vi "Update Controller State.vi"(8 "error in (no error)":errorcluster, 11 "Elevator Controller Actor in":refnum<class "Elevator Controller Actor.lvclass">) -> (0 "error out":errorcluster, 3 "Elevator Controller Actor out":refnum<class "Elevator Controller Actor.lvclass">)   [LabVIEW 2019, in "Elevator Controller Actor.lvlib" / "Elevator Controller Actor.lvclass"]
uses:
  Elevator Controller Actor.lvclass
  <vilib>/ActorFramework/Actor/Actor.lvclass
  Sim Display Console Actor/Elevator Controller/Elevator Direction.ctl
  Sim Display Console Actor/Elevator Controller/Sim Display Console Actor.lvclass
  Elevator Controller Actor Messages/Set State Msg/Set State Msg.lvclass
  State -Enum.ctl
  Sim User Console Actor/Elevator Controller/Floor Selection.ctl
  Sim User Console Actor/Elevator Controller/Sim User Console Actor.lvclass
  Sim User Console Actor/Elevator Controller/Elevator Call.ctl
  Sim Display Console Actor/Elevator Controller/Floor -Enum.ctl
  Configuration Database Actor/Configuration Database Actor Messages/Read Record(sec) Msg/Read Record(sec) Msg.lvclass
  Configuration Database Actor/Configuration Database Actor Messages/Write Record(sec) Msg/Write Record(sec) Msg.lvclass
  <vilib>/ActorFramework/Message Enqueuer/Message Enqueuer.lvclass
  Configuration Database Actor/Configuration Database Actor/Record -Cluster.ctl
  Configuration Database Actor/Configuration Database Actor/Configuration Database Actor.lvclass
  Sim Display Console Actor/Sim Display Console Actor Messages/Read value elevator location Msg/Read value elevator location Msg.lvclass
  Sim Display Console Actor/Sim Display Console Actor Messages/Write Timing Msg/Write Timing Msg.lvclass
  Sim User Console Actor/Sim User Console Actor Messages/Disable Doors Msg/Disable Doors Msg.lvclass
  Simulated Sensor Interface Actor/Sim Sensor Interface Messages/Write Elevator Position Msg/Write Elevator Position Msg.lvclass
  Sim Display Console Actor/Sim Display Console Actor Messages/Write Elevator Location Msg/Write Elevator Location Msg.lvclass
  Sim Display Console Actor/Sim Display Console Actor Messages/Write Elevator Direction Msg/Write Elevator Direction Msg.lvclass
  Sim Display Console Actor/Sim Display Console Actor Messages/Write Door Open Msg/Write Door Open Msg.lvclass
  Sim Display Console Actor/Sim Display Console Actor Messages/Write Emergency Ind Msg/Write Emergency Ind Msg.lvclass
  Sim User Console Actor/Sim User Console Actor Messages/Write Elevator Call Msg/Write Elevator Call Msg.lvclass
  Sim User Console Actor/Sim User Console Actor Messages/Write Doors Msg/Write Doors Msg.lvclass
  Sim User Console Actor/Elevator Controller/Door Buttons.ctl
  Sim User Console Actor/Sim User Console Actor Messages/Write Floor Selection Msg/Write Floor Selection Msg.lvclass
  Sim User Console Actor/Sim User Console Actor Messages/Write Emergency Msg/Write Emergency Msg.lvclass
  Sim User Console Actor/Sim User Console Actor Messages/Read all Controls Msg/Read all Controls Msg.lvclass
  Sim Display Console Actor/Sim Display Console Actor Messages/Read Elevator Direction Msg/Read Elevator Direction Msg.lvclass
  Elevator Controller Actor Messages/Set Enable Door Msg/Set Enable Door Msg.lvclass
  Sim User Console Actor/Sim User Console Actor Messages/Disable All components Msg/Disable All components Msg.lvclass
  C:/Program Files (x86)/National Instruments/LabVIEW 2019/vi.lib/ActorFramework/Actor/Actor.lvclass
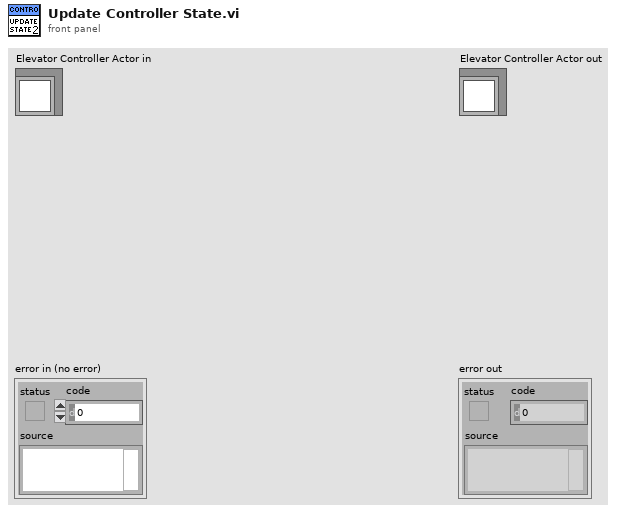
[diagram p1: front panel]
types:
  T1 = typedef "Simulated User Console Actor.lvlib/Sim User Console Actor.lvclass/Floor Selection.ctl" = cluster{"Floor4":bool, "Floor 3":bool, "Floor2":bool, "Floor1":bool}
  T2 = typedef "Simulated User Console Actor.lvlib/Sim User Console Actor.lvclass/Door Buttons.ctl" = cluster{"Open Door":bool, "Close Door":bool}
  T3 = typedef "Simulated User Console Actor.lvlib/Sim User Console Actor.lvclass/Elevator Call.ctl" = cluster{"Up":bool, "Up 2":bool, "Up 3":bool, "Down":bool, "Down 2":bool, "Down 3":bool}
  T4 = typedef "Simulated Display Console Actor.lvlib/Sim Display Console Actor.lvclass/Elevator Direction.ctl" = cluster{"Up":bool, "Down":bool}
  T5 = typedef "Simulated Display Console Actor.lvlib/Sim Display Console Actor.lvclass/Floor -Enum.ctl" = enum16{"First Floor", "Send Floor", "Third Floor", "Fourth Floor"}
  T6 = typedef "Configuration Database Actor.lvlib/Configuration Database Actor.lvclass/Record -Cluster.ctl" = cluster{"Door Open":dbl, "Door close":dbl, "Travel Time":dbl, "Inactive Time":dbl}
  T7 = enum8{"Enabled", "Disabled", "Disabled and Grayed Out"}
  T8 = typedef "Elevator Controller Actor.lvlib/Elevator Controller Actor.lvclass/State -Enum.ctl" = enum16{"Initial", "Wait for First Request", "Start and Move", "Anaysis", "Continue Travel", "Stop at Floor", "Open and Close Door Sequence", "No Request Remaining", "Emergency Call", "Terminate Process"}
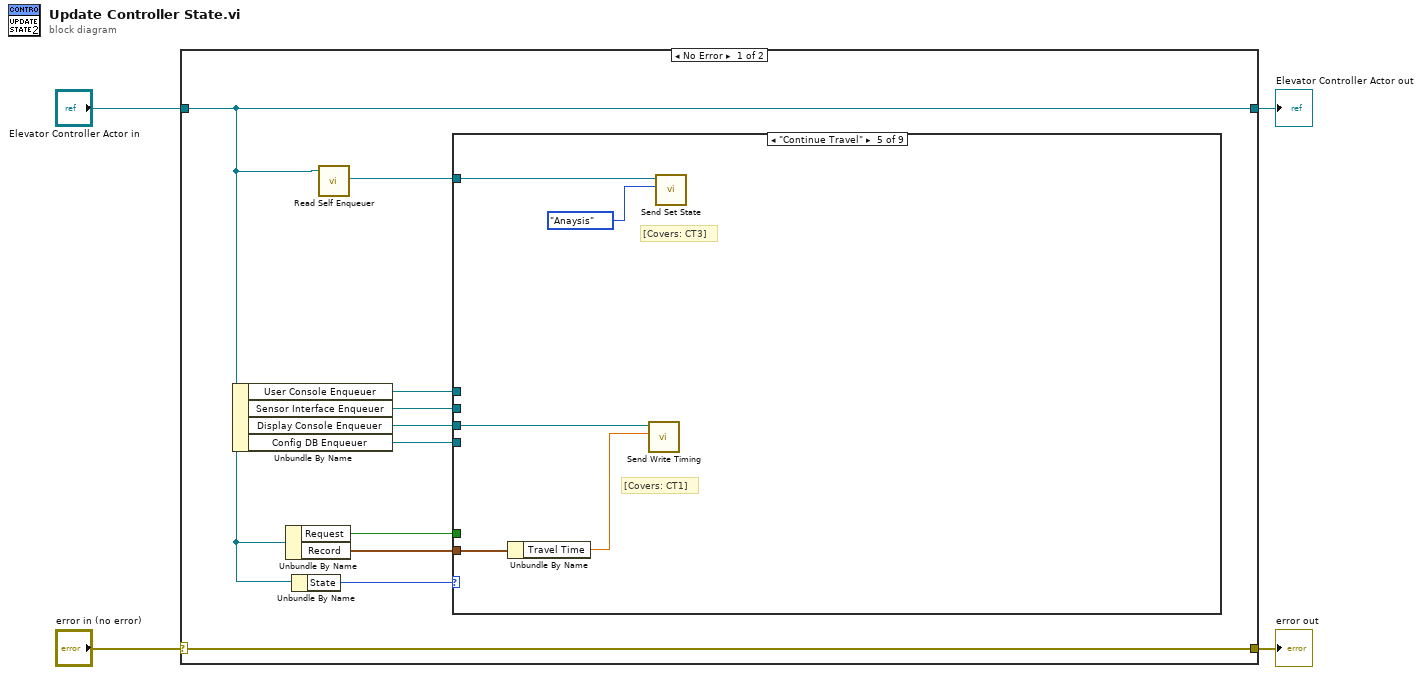
[diagram p0: block diagram]
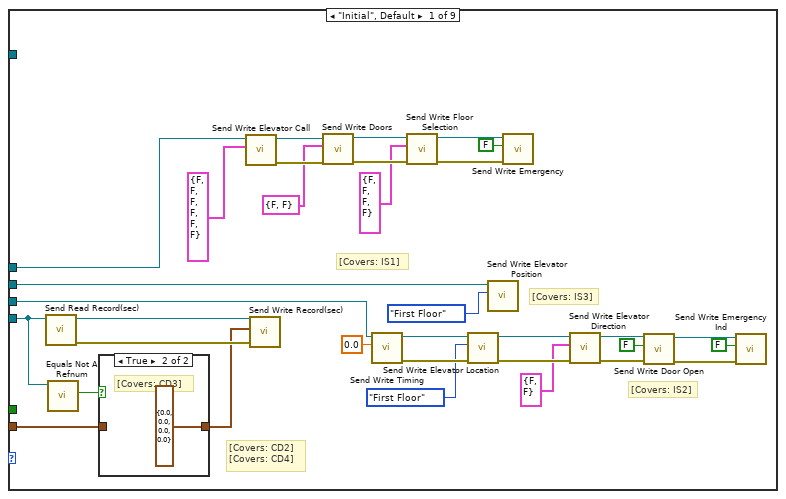
[diagram p2: hidden frame]
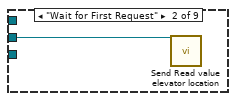
[diagram p4: hidden frame]
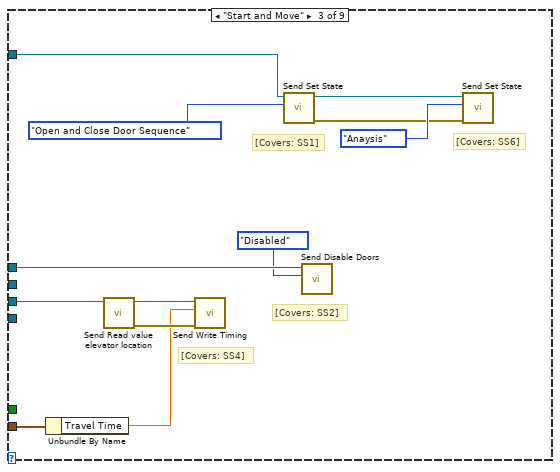
[diagram p5: hidden frame]
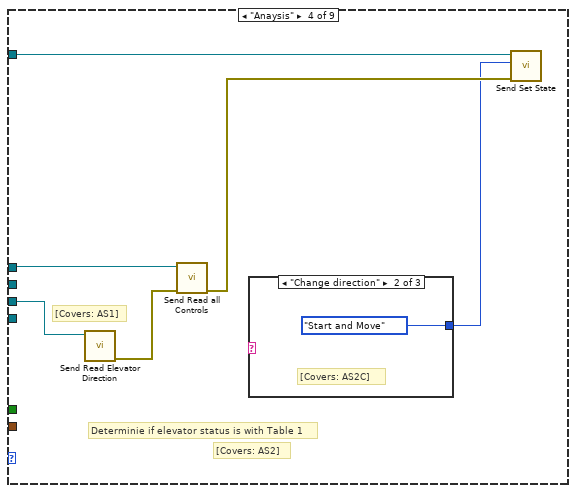
[diagram p6: hidden frame]
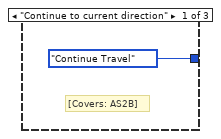
[diagram p7: hidden frame]
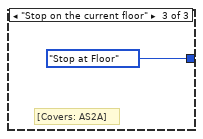
[diagram p8: hidden frame]
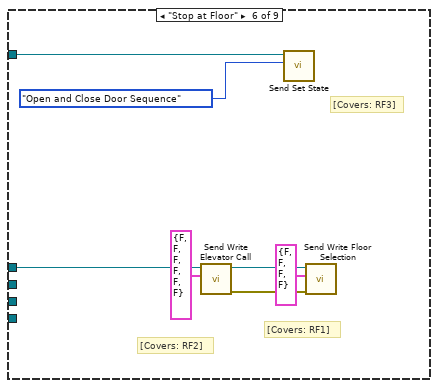
[diagram p9: hidden frame]
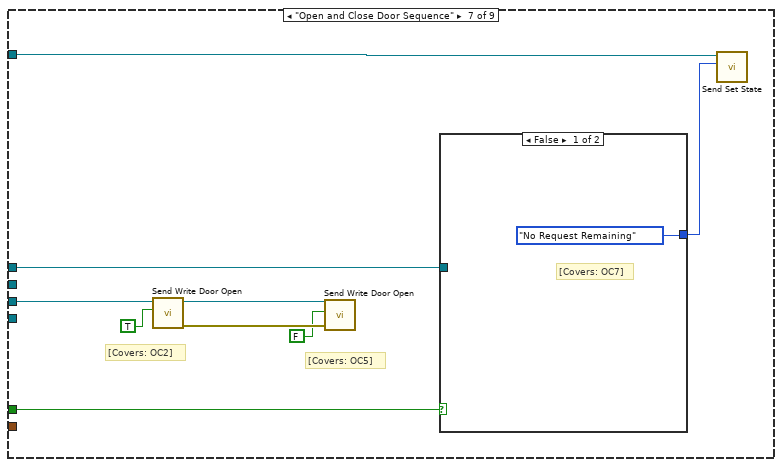
[diagram p10: hidden frame]
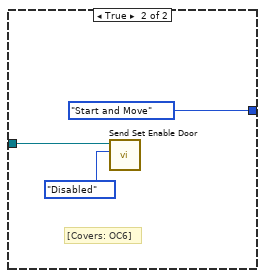
[diagram p11: hidden frame]
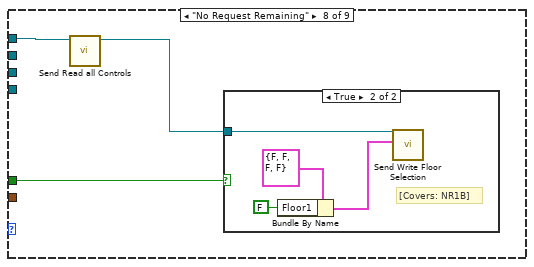
[diagram p12: hidden frame]
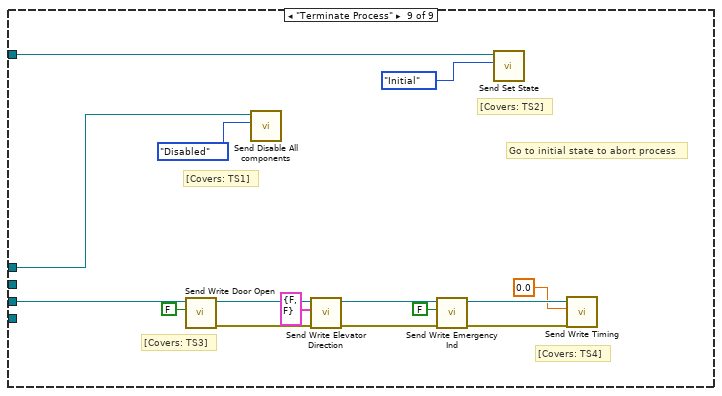
[diagram p14: hidden frame]
diagram:
  n1 = case shown="No Error" "error in (no error)" {
    selector: "error in (no error)" -> [w14 w120]
    tunnel: [w14 w120] -> w3
    tunnel: [w10 w119] -> w1
    tunnel: "Elevator Controller Actor in" -> [w10 w119]
    frame No Error {
      n2 = Unbundle By Name(w10) -> ("User Console Enqueuer"=w6:refnum<class "Message Enqueuer.lvclass">, "Sensor Interface Enqueuer"=w7:refnum<class "Message Enqueuer.lvclass">, "Display Console Enqueuer"=w8:refnum<class "Message Enqueuer.lvclass">, "Config DB Enqueuer"=w11:refnum<class "Message Enqueuer.lvclass">)
      n3 = Unbundle By Name(w10) -> ("Request"=w5:bool, "Record"=w9:T6)
      n4 = Unbundle By Name(w10) -> ("State"=w13:T8)
      n5 = call <vilib>:"Read Self Enqueuer.vi"("Actor"=w10) -> ("Self Enqueuer"=w12:refnum<class "Message Enqueuer.lvclass">)  [unwired: 10 in]
      n6 = case shown="\"Continue Travel\"" w13 {
        tunnel: w12 -> [_ _ w61 w65 w75 w83 w92 _ w105]
        tunnel: w11 -> [w45 _ _ _ _ _ _ _ _]
        tunnel: w9 -> [w43 _ w57 _ w74 _ _ _ _]
        tunnel: w8 -> [w39 w50 w58 w67 w73 _ w91 _ w116]
        tunnel: w7 -> [w40 _ _ _ _ _ _ _ _]
        tunnel: w6 -> [w25 _ w52 w68 _ w79 w85 w98 w118]
        tunnel: w5 -> [_ _ _ _ _ _ w86 w99 _]
        frame "Initial", Default {
          # "[Covers: CD2] \n[Covers: CD4]"
          # "[Covers: IS3]"
          # "[Covers: IS2]"
          # "[Covers: IS1]"
          n7 = call "Send Read Record(sec).vi"("Message Enqueuer"=w45) -> ("error out"=w46:errorcluster, "Message Enqueuer out"=w47:refnum<class "Message Enqueuer.lvclass">)  [unwired: 9 in]
          n8 = call <vilib>:"Equals Not A Refnum.vi"("Message Enqueuer"=w45) -> ("Not a refnum?"=w44:bool)  [unwired: 10 in]
          n9 = case shown="True" w44 {
            tunnel: [w48 T6 {"Door Open"=0.0, "Door close"=0.0, "Travel Time"=0.0, "Inactive Time"=0.0} ("Record")] -> w42
            tunnel: w43 -> [w48 _]
            frame False {
            }
            frame True {
              # "[Covers: CD3]"
            }
          }
          n10 = call "Send Write Elevator Call.vi"("Elevator Call"=T3 {"Up"=FALSE, "Up 2"=FALSE, "Up 3"=FALSE, "Down"=FALSE, "Down 2"=FALSE, "Down 3"=FALSE}, "Message Enqueuer"=w25) -> ("error out"=w23:errorcluster, "Message Enqueuer out"=w22:refnum<class "Message Enqueuer.lvclass">)  [unwired: 8 in]
          n11 = call "Send Write Record(sec).vi"("error in (no error)"=w46, "Record"=w42, "Message Enqueuer"=w47) -> ()  [unwired: 7 in, 2 out]
          n12 = call "Send Write Doors.vi"("error in (no error)"=w23, "Doors"=T2 {"Open Door"=FALSE, "Close Door"=FALSE}, "Message Enqueuer"=w22) -> ("error out"=w19:errorcluster, "Message Enqueuer out"=w20:refnum<class "Message Enqueuer.lvclass">)  [unwired: 7 in]
          n13 = call "Send Write Timing.vi"("Time"=0.0, "Message Enqueuer"=w39) -> ("error out"=w36:errorcluster, "Message Enqueuer out"=w37:refnum<class "Message Enqueuer.lvclass">)  [unwired: 8 in]
          n14 = call "Send Write Floor Selection.vi"("error in (no error)"=w19, "Floor Selection"=T1 {"Floor4"=FALSE, "Floor 3"=FALSE, "Floor2"=FALSE, "Floor1"=FALSE}, "Message Enqueuer"=w20) -> ("error out"=w17:errorcluster, "Message Enqueuer out"=w16:refnum<class "Message Enqueuer.lvclass">)  [unwired: 7 in]
          n15 = call "Send Write Elevator Location.vi"("error in (no error)"=w36, "Elevator Location"=Floor_-Enum."First Floor", "Message Enqueuer"=w37) -> ("error out"=w33:errorcluster, "Message Enqueuer out"=w34:refnum<class "Message Enqueuer.lvclass">)  [unwired: 7 in]
          n16 = call "Send Write Elevator Position.vi"("Elevator Position"=Floor_-Enum."First Floor" ("Floor"), "Message Enqueuer"=w40) -> ()  [unwired: 8 in, 2 out]
          n17 = call "Send Write Emergency.vi"("error in (no error)"=w17, "Emergenc"=FALSE, "Message Enqueuer"=w16) -> ()  [unwired: 7 in, 2 out]
          n18 = call "Send Write Elevator Direction.vi"("error in (no error)"=w33, "Elevator Direction"=T4 {"Up"=FALSE, "Down"=FALSE}, "Message Enqueuer"=w34) -> ("error out"=w30:errorcluster, "Message Enqueuer out"=w31:refnum<class "Message Enqueuer.lvclass">)  [unwired: 7 in]
          n19 = call "Send Write Door Open.vi"("error in (no error)"=w30, "Door Open"=FALSE, "Message Enqueuer"=w31) -> ("error out"=w28:errorcluster, "Message Enqueuer out"=w27:refnum<class "Message Enqueuer.lvclass">)  [unwired: 7 in]
          n20 = call "Send Write Emergency Ind.vi"("error in (no error)"=w28, "Emergency"=FALSE, "Message Enqueuer"=w27) -> ()  [unwired: 7 in, 2 out]
        }
        frame "Wait for First Request" {
          n21 = call "Send Read value elevator location.vi"("Message Enqueuer"=w50) -> ()  [unwired: 9 in, 2 out]
        }
        frame "Start and Move" {
          # "[Covers: SS1]"
          # "[Covers: SS4]"
          # "[Covers: SS6]"
          # "[Covers: SS2]"
          n22 = Unbundle By Name(w57) -> ("Travel Time"=w54:dbl)
          n23 = call "Send Read value elevator location.vi"("Message Enqueuer"=w58) -> ("error out"=w56:errorcluster, "Message Enqueuer out"=w55:refnum<class "Message Enqueuer.lvclass">)  [unwired: 9 in]
          n24 = call "Send Write Timing.vi"("error in (no error)"=w56, "Time"=w54, "Message Enqueuer"=w55) -> ()  [unwired: 7 in, 2 out]
          n25 = call "Send Set State.vi"("States"=State_-Enum."Open and Close Door Sequence", "Message Enqueuer"=w61) -> ("error out"=w59:errorcluster, "Message Enqueuer out"=w53:refnum<class "Message Enqueuer.lvclass">)  [unwired: 8 in]
          n26 = call "Send Disable Doors.vi"("Disabled"=T7."Disabled", "Message Enqueuer"=w52) -> ()  [unwired: 8 in, 2 out]
          n27 = call "Send Set State.vi"("error in (no error)"=w59, "States"=State_-Enum."Anaysis", "Message Enqueuer"=w53) -> ()  [unwired: 7 in, 2 out]
        }
        frame "Anaysis" {
          # "[Covers: AS2]"
          # "Determinie if elevator status is with Table 1"
          # "[Covers: AS1]"
          n28 = call "Send Read Elevator Direction.vi"("Message Enqueuer"=w67) -> ("error out"=w66:errorcluster)  [unwired: 9 in, 1 out]
          n29 = call "Send Read all Controls.vi"("error in (no error)"=w66, "Message Enqueuer"=w68) -> ("error out"=w64:errorcluster)  [unwired: 8 in, 1 out]
          n30 = case shown="\"Change direction\"" {
            selector: _ -> [_ _ _]
            tunnel: [State_-Enum."Continue Travel" ("States") State_-Enum."Start and Move" ("States") State_-Enum."Stop at Floor" ("States")] -> w63
            frame "Continue to current direction" {
              # "[Covers: AS2B]"
            }
            frame "Change direction" {
              # "[Covers: AS2C]"
            }
            frame "Stop on the current floor" {
              # "[Covers: AS2A]"
            }
          }
          n31 = call "Send Set State.vi"("error in (no error)"=w64, "States"=w63, "Message Enqueuer"=w65) -> ()  [unwired: 7 in, 2 out]
        }
        frame "Continue Travel" {
          # "[Covers: CT1]"
          # "[Covers: CT3]"
          n32 = Unbundle By Name(w74) -> ("Travel Time"=w72:dbl)
          n33 = call "Send Write Timing.vi"("Time"=w72, "Message Enqueuer"=w73) -> ()  [unwired: 8 in, 2 out]
          n34 = call "Send Set State.vi"("States"=State_-Enum."Anaysis", "Message Enqueuer"=w75) -> ()  [unwired: 8 in, 2 out]
        }
        frame "Stop at Floor" {
          # "[Covers: RF3]"
          # "[Covers: RF2]"
          # "[Covers: RF1]"
          n35 = call "Send Write Elevator Call.vi"("Elevator Call"=T3 {"Up"=FALSE, "Up 2"=FALSE, "Up 3"=FALSE, "Down"=FALSE, "Down 2"=FALSE, "Down 3"=FALSE}, "Message Enqueuer"=w79) -> ("error out"=w80:errorcluster, "Message Enqueuer out"=w81:refnum<class "Message Enqueuer.lvclass">)  [unwired: 8 in]
          n36 = call "Send Set State.vi"("States"=State_-Enum."Open and Close Door Sequence", "Message Enqueuer"=w83) -> ()  [unwired: 8 in, 2 out]
          n37 = call "Send Write Floor Selection.vi"("error in (no error)"=w80, "Floor Selection"=T1 {"Floor4"=FALSE, "Floor 3"=FALSE, "Floor2"=FALSE, "Floor1"=FALSE}, "Message Enqueuer"=w81) -> ()  [unwired: 7 in, 2 out]
        }
        frame "Open and Close Door Sequence" {
          # "[Covers: OC5]"
          # "[Covers: OC2]"
          n38 = call "Send Write Door Open.vi"("Door Open"=TRUE, "Message Enqueuer"=w91) -> ("error out"=w88:errorcluster, "Message Enqueuer out"=w89:refnum<class "Message Enqueuer.lvclass">)  [unwired: 8 in]
          n39 = call "Send Write Door Open.vi"("error in (no error)"=w88, "Door Open"=FALSE, "Message Enqueuer"=w89) -> ()  [unwired: 7 in, 2 out]
          n40 = case shown="False" w86 {
            tunnel: w85 -> [_ w96]
            tunnel: [State_-Enum."No Request Remaining" ("States") State_-Enum."Start and Move" ("States")] -> w84
            frame False {
              # "[Covers: OC7]"
            }
            frame True {
              # "[Covers: OC6]"
              n41 = call "Send Set Enable Door.vi"("Disabled"=T7."Disabled", "Message Enqueuer"=w96) -> ()  [unwired: 8 in, 2 out]
            }
          }
          n42 = call "Send Set State.vi"("States"=w84, "Message Enqueuer"=w92) -> ()  [unwired: 8 in, 2 out]
        }
        frame "No Request Remaining" {
          n43 = call "Send Read all Controls.vi"("Message Enqueuer"=w98) -> ("Message Enqueuer out"=w97:refnum<class "Message Enqueuer.lvclass">)  [unwired: 9 in, 1 out]
          n44 = case shown="True" w99 {
            tunnel: w97 -> [_ w103]
            frame False {
            }
            frame True {
              # "[Covers: NR1B]"
              n45 = Bundle By Name(cluster=T1 {"Floor4"=FALSE, "Floor 3"=FALSE, "Floor2"=FALSE, "Floor1"=FALSE} ("Floor Selection"), "Floor1"=FALSE) -> (w101:T1)
              n46 = call "Send Write Floor Selection.vi"("Floor Selection"=w101, "Message Enqueuer"=w103) -> ()  [unwired: 8 in, 2 out]
            }
          }
        }
        frame "Terminate Process" {
          # "[Covers: TS3]"
          # "[Covers: TS4]"
          # "Go to initial state to abort process"
          # "[Covers: TS2]"
          # "[Covers: TS1]"
          n47 = call "Send Write Door Open.vi"("Door Open"=FALSE, "Message Enqueuer"=w116) -> ("error out"=w114:errorcluster, "Message Enqueuer out"=w115:refnum<class "Message Enqueuer.lvclass">)  [unwired: 8 in]
          n48 = call "Send Disable All components.vi"("Disabled"=T7."Disabled", "Message Enqueuer"=w118) -> ()  [unwired: 8 in, 2 out]
          n49 = call "Send Write Elevator Direction.vi"("error in (no error)"=w114, "Elevator Direction"=T4 {"Up"=FALSE, "Down"=FALSE}, "Message Enqueuer"=w115) -> ("error out"=w113:errorcluster, "Message Enqueuer out"=w112:refnum<class "Message Enqueuer.lvclass">)  [unwired: 7 in]
          n50 = call "Send Write Emergency Ind.vi"("error in (no error)"=w113, "Emergency"=FALSE, "Message Enqueuer"=w112) -> ("error out"=w108:errorcluster, "Message Enqueuer out"=w107:refnum<class "Message Enqueuer.lvclass">)  [unwired: 7 in]
          n51 = call "Send Set State.vi"("States"=State_-Enum."Initial", "Message Enqueuer"=w105) -> ()  [unwired: 8 in, 2 out]
          n52 = call "Send Write Timing.vi"("error in (no error)"=w108, "Time"=0.0, "Message Enqueuer"=w107) -> ()  [unwired: 7 in, 2 out]
        }
      }
    }
    frame Error {
    }
  }
  "error out" <- w3
  "Elevator Controller Actor out" <- w1
